vi "Write ACIR Setting.vi"(8 "error in (no error)":errorcluster, 10 "ACIR Setting":T1={"DC Voltage"=0.0, "High Limit"=100000.0, "Test Time(s)"=100000} {"High Limit" format="%#_6f"; "DC Voltage" format="%#_6f"}, 11 "ACIR configuration":refnum<class "HiPOT configuration.lvclass">) -> (0 "error out":errorcluster, 3 "ACIR configuration out":refnum<class "HiPOT configuration.lvclass">)   [LabVIEW 2025, in "HiPOT.lvlib" / "HiPOT configuration.lvclass"]
uses:
  HiPOT configuration.lvclass
  HiPOT Instrument Setting.ctl
  HiPOT configuration.lvclass/HiPOT configuration.ctl
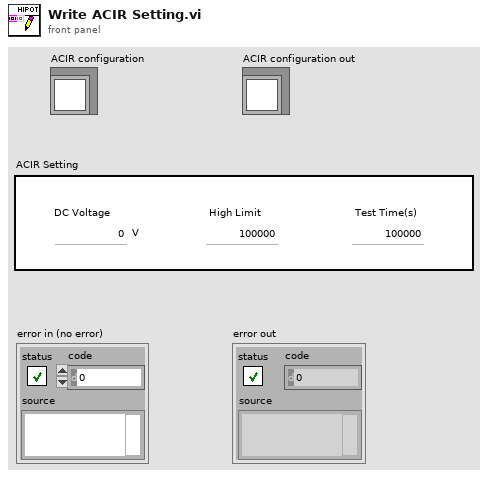
[diagram p1: front panel]
types:
  T1 = typedef "HiPOT.lvlib/HiPOT configuration.lvclass/HiPOT Instrument Setting.ctl" = cluster{"DC Voltage":dbl, "High Limit":dbl, "Test Time(s)":u32}
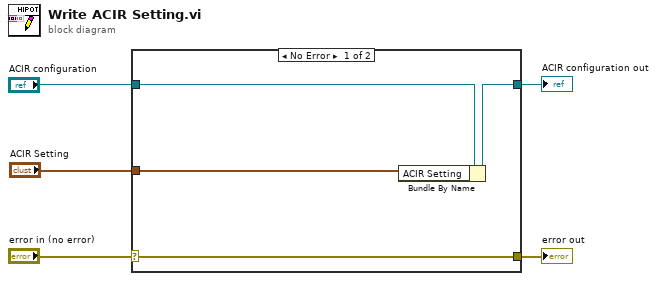
[diagram p0: block diagram]
diagram:
  n1 = case shown="No Error" "error in (no error)" {
    selector: "error in (no error)" -> [w9 w10]
    tunnel: [w9 w10] -> w4
    tunnel: [w7 w11] -> w2
    tunnel: "ACIR configuration" -> [w8 w11]
    tunnel: "ACIR Setting" -> [w6 _]
    frame No Error {
      n2 = Bundle By Name(cluster=w8, "ACIR Setting"=w6) -> (w7:refnum<class "HiPOT configuration.lvclass">)
    }
    frame Error {
    }
  }
  "error out" <- w4
  "ACIR configuration out" <- w2
